vi "DeleteUser.vi"(8 "error in (no error)":errorcluster) -> (0 "error out":errorcluster)   [LabVIEW 2021]
panel:
  in  "Select User":string(combo)
  in  "Delete User":bool
  in  "Cancel":bool
  in  "Help":bool
  # "Delete User"
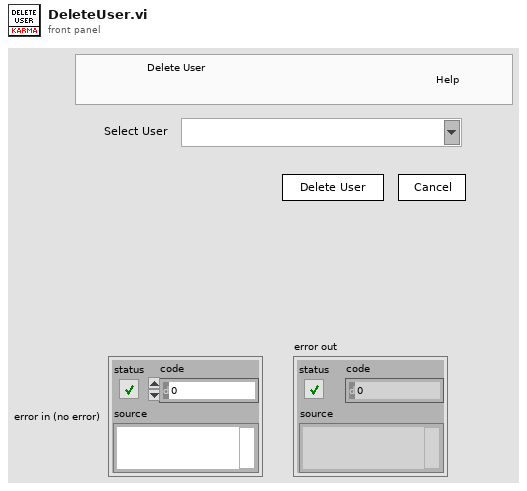
[diagram p1: front panel]
types:
  T1 = enum16{"Poll", "Initialize", "DeleteUser", "Error", "Exit"}
  T2 = typedef "UserInfo.ctl" = cluster{"User Name":string, "Password":string, "UserType":T3}
  T3 = typedef "UserTypes.ctl" = u16
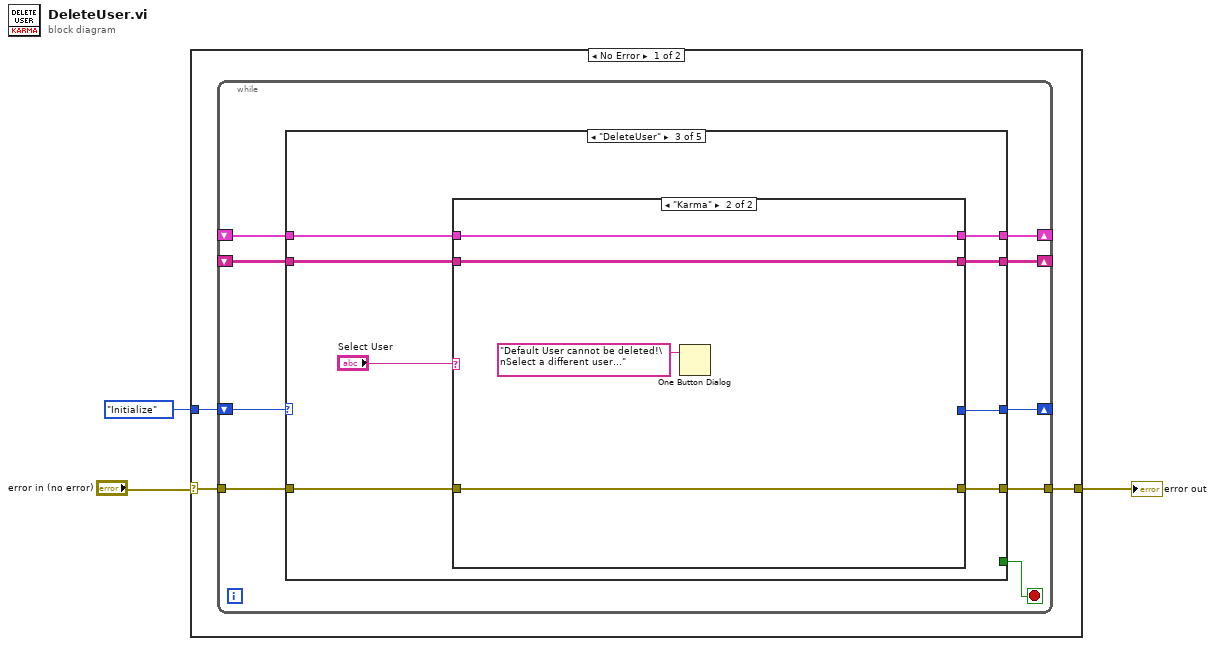
[diagram p0: block diagram]
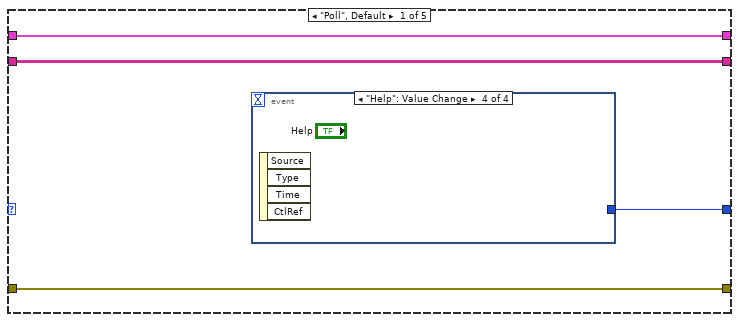
[diagram p2: hidden frame]
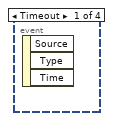
[diagram p3: hidden frame]
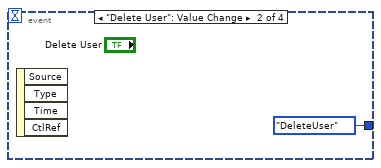
[diagram p4: hidden frame]
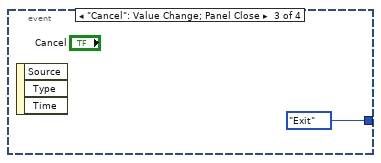
[diagram p5: hidden frame]
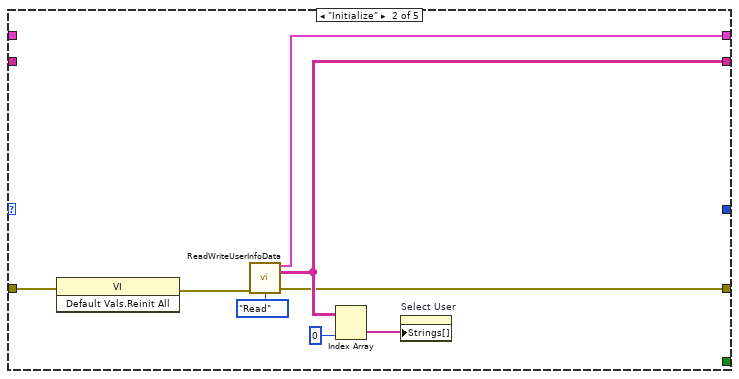
[diagram p6: hidden frame]
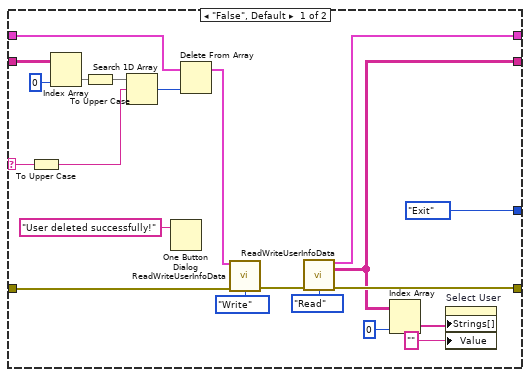
[diagram p7: hidden frame]
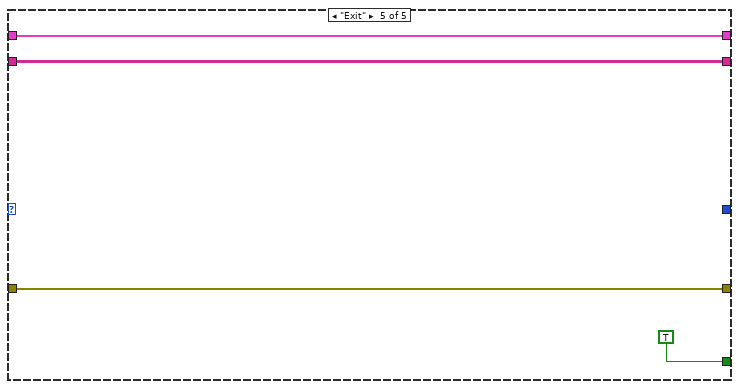
[diagram p9: hidden frame]
diagram:
  n1 = case shown="No Error" "error in (no error)" {
    selector: "error in (no error)" -> [w6 w70]
    tunnel: T1."Initialize" -> [w5 _]
    tunnel: [w4 w70] -> w2
    frame No Error {
      n2 = while {
        tunnel: w6 -> [w15]
        shift-right: [w13] -> _
        shift-left: w5 -> [w14]
        shift-right: [w12] -> _
        shift-left: _ -> [w11]
        shift-right: [w10] -> _
        shift-left: _ -> [w9]
        tunnel: [w8] -> w4
        stop <- w7 stop-if-true
        n3 = case shown="\"DeleteUser\"" w14 {
          tunnel: w15 -> [w18 w29 w33 w65 w67]
          tunnel: [w19 _ w30 _ _] -> w13
          tunnel: [w16 w25 w34 w63 w68] -> w12
          tunnel: w11 -> [w16 _ w36 w63 w68]
          tunnel: [w17 w24 w35 w64 w69] -> w10
          tunnel: w9 -> [w17 _ w37 w64 w69]
          tunnel: [w18 w23 w32 w65 w67] -> w8
          tunnel: [_ _ _ _ TRUE] -> w7
          frame "Poll", Default {
            n4 = event shown="[3] \"Help\": Value Change" {
              selector: _ -> [_ _ _ _]
              dyn-events: _ -> [_ _ _ _]
              timeout: _ -> [_ _ _ _]
              tunnel: [_ T1."DeleteUser" T1."Exit" _] -> w19
              event Timeout {
                n5 = event-data() -> ()  [unwired: 1 in, 3 out]
              }
              event "Delete User": Value Change {
                n6 = event-data() -> ()  [unwired: 1 in, 4 out]
              }
              event "Cancel": Value Change; Panel Close {
                n7 = event-data() -> ()  [unwired: 1 in, 3 out]
              }
              event "Help": Value Change {
                n8 = event-data() -> ()  [unwired: 1 in, 4 out]
              }
            }
          }
          frame "Initialize" {
            n9 = invoke class="VI" method="Default Vals.Reinit All"(error in=w29) -> (error out=w26:errorcluster)  [unwired: 2 in, 2 out]
            n10 = call "ReadWriteUserInfoData.vi"("Error in (no error)"=w26, "Operation"=enum16{"Write", "Read"}."Read") -> ("User Info Array of Clusters Out"=w24:T2[], "User Info Array out"=w25:string[][], "Error out"=w23:errorcluster)  [unwired: 11 in]
            n11 = Index Array(array=w25, index (col)=0 ("disabled index (col)")) -> (element=w22:string[])  [unwired: 1 in]
            n12 = property on="Select User" class="CmbBox"("Strings[]"=w22) -> ()  [unwired: 2 in, 2 out]
          }
          frame "DeleteUser" {
            n13 = case shown="\"Karma\"" "Select User" {
              selector: "Select User" -> [w54 _]
              tunnel: w37 -> [w52 w62]
              tunnel: w36 -> [w58 w61]
              tunnel: [w44 w62] -> w35
              tunnel: [w42 w61] -> w34
              tunnel: w33 -> [w49 w60]
              tunnel: [w46 w60] -> w32
              tunnel: [T1."Exit" _] -> w30
              frame "False", Default {
                n14 = To Upper Case(1:w54) -> (0:w53:string)
                n15 = Index Array(array=w58, index (col)=0 ("disabled index (col)")) -> (element=w56:string[])  [unwired: 1 in]
                n16 = To Upper Case(1:w56) -> (0:w55:string[])
                n17 = Search 1D Array(1D array=w55, element=w53) -> (index of element=w51:i32)  [unwired: 1 in]
                n18 = One Button Dialog(message="User deleted successfully!") -> ()  [unwired: 1 in, 1 out]
                n19 = Delete From Array(array=w52, index=w51) -> (array with subset deleted=w50:T2[])  [unwired: 1 in, 1 out]
                n20 = call "ReadWriteUserInfoData.vi"("User Info  Array In"=w50, "Error in (no error)"=w49, "Operation"=enum16{"Write", "Read"}."Write") -> ("Error out"=w47:errorcluster)  [unwired: 10 in, 2 out]
                n21 = call "ReadWriteUserInfoData.vi"("Error in (no error)"=w47, "Operation"=enum16{"Write", "Read"}."Read") -> ("User Info Array of Clusters Out"=w44:T2[], "User Info Array out"=w42:string[][], "Error out"=w46:errorcluster)  [unwired: 11 in]
                n22 = Index Array(array=w42, index (col)=0 ("disabled index (col)")) -> (element=w40:string[])  [unwired: 1 in]
                n23 = property on="Select User" class="CmbBox"("Strings[]"=w40, "Value"="") -> ()  [unwired: 2 in, 2 out]
              }
              frame "Karma" {
                n24 = One Button Dialog(message="Default User cannot be deleted!\nSelect a different user...") -> ()  [unwired: 1 in, 1 out]
              }
            }
          }
          frame "Error" {
          }
          frame "Exit" {
          }
        }
      }
    }
    frame Error {
    }
  }
  "error out" <- w2
